vi "Check Path Availability.vi"(8 "error in (no error)":errorcluster, 9 "channel 2":string, 10 "channel 1":string, 11 "Route Manager in":refnum<class "Route Manager.lvclass">) -> (0 "error out":errorcluster, 2 "path capability":T1=1 items=["Path Available"=1, "Path Exists"=2, "Path Unsupported"=3, "Resource in Use"=4, "Source Conflict"=5, "Channel Not Available"=6])   [LabVIEW 2015, in "Route Manager.lvclass"]
uses:
  Route Manager.lvclass
  SLSC Switch/Path Capability.ctl
  SLSC Switch/SLSC Switch.lvclass
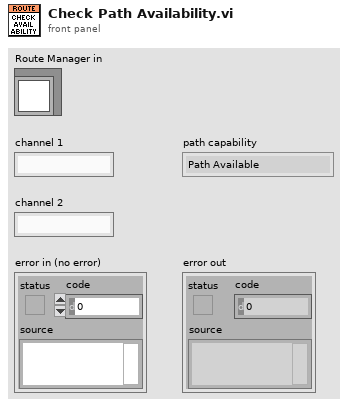
[diagram p1: front panel]
types:
  T1 = typedef "SLSC Switch.lvclass/Path Capability.ctl" = i32
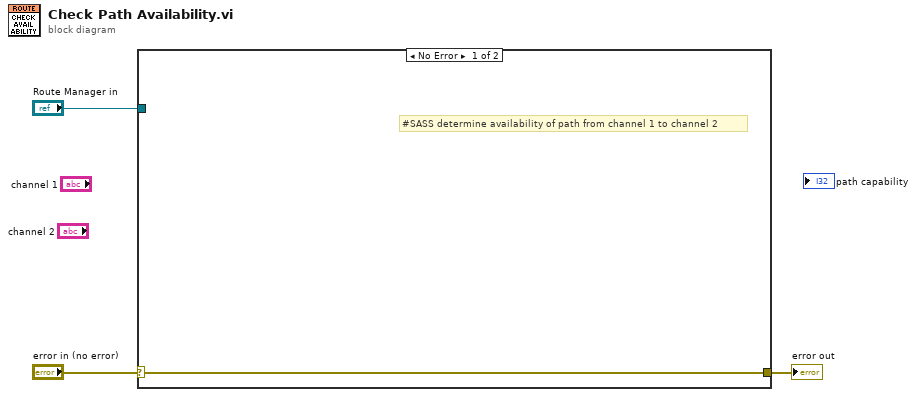
[diagram p0: block diagram]
diagram:
  n1 = case shown="No Error" "error in (no error)" {
    selector: "error in (no error)" -> [w4 w5]
    tunnel: [w4 w5] -> w2
    tunnel: "Route Manager in" -> [_ _]
    frame No Error {
      # "#SASS determine availability of path from channel 1 to channel 2"
    }
    frame Error {
    }
  }
  "error out" <- w2
